vi "Serial Read.vi"(9 "Timeout (ms)":i32, 10 "Number of Bytes to Read":u32, 11 "IO Cluster In":T1={"Error"={"status"=FALSE, "code"=0, "source"=""}, "Encoder Calibration Values"=[22, 216], "Update Calibration"=FALSE, "JPEG Resolutions"=3, "Raw Resolutions"=1, "Image Mode"=enum."RAW Gray Scale", "FPGA Ref"=refnum} {"JPEG Resolutions" items=["160x128"=3, "320x240"=5, "640x480"=7]; "Raw Resolutions" items=["80x60"=1, "160x120"=3, "128x128"=9, "128x96"=11]}) -> (1 "Data Valid":bool, 2 "Data":u8[](array[numeric]), 3 "IO Cluster Out":T1={"Error"={"status"=FALSE, "code"=0, "source"=""}, "Encoder Calibration Values"=[22, 216], "Update Calibration"=FALSE, "JPEG Resolutions"=3, "Raw Resolutions"=1, "Image Mode"=enum."RAW Gray Scale", "FPGA Ref"=refnum} {"JPEG Resolutions" items=["160x128"=3, "320x240"=5, "640x480"=7]; "Raw Resolutions" items=["80x60"=1, "160x120"=3, "128x128"=9, "128x96"=11]}, 4 "Framing Error":bool, 6 "Bytes in Buffer":u32)   [LabVIEW 2019]
uses:
  QNET MS IO Cluster.ctl
  <vilib>/Utility/error.llb/Error Cluster From Error Code.vi
  <vilib>/rvi/errors/niLvFpgaAdjustHostInterfaceError.vi
  <vilib>/rvi/interface/nirviMethod/nirviMethod.xnode
  <vilib>/rvi/interface/nirviReadWriteControl/nirviReadWriteControl.xnode
  <vilib>/FPGAPlugInAG/Dynamic/niLvFpga_ReadFifo_Dynamic.vi
  <vilib>/rvi/errors/niLvFpgaMergeErrorWithErrorCode.vi
  NiFpgaLv.dll
  <vilib>/rvi/interface/Simulation/niFpgaSimulationCallBeginRW.vi
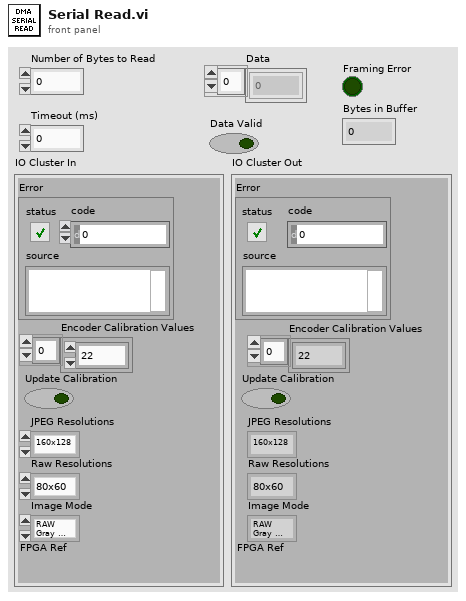
[diagram p1: front panel]
types:
  T1 = typedef "QNET MS IO Cluster.ctl" = cluster{"Error":errorcluster, "Encoder Calibration Values":i32[], "Update Calibration":bool, "JPEG Resolutions":u16, "Raw Resolutions":u16, "Image Mode":enum16{"RAW RGB", "RAW Gray Scale", "JPEG"}, "FPGA Ref":refnum<k20>}
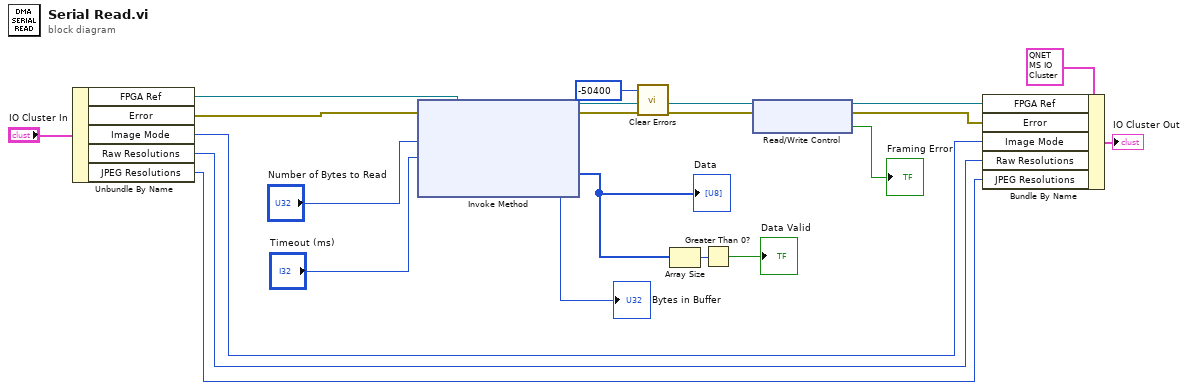
[diagram p0: block diagram]
diagram:
  n1 = Unbundle By Name("IO Cluster In") -> ("FPGA Ref"=w13:refnum<k20>, "Error"=w12:errorcluster, "Image Mode"=w9:enum16{"RAW RGB", "RAW Gray Scale", "JPEG"}, "Raw Resolutions"=w8:u16, "JPEG Resolutions"=w7:u16)
  n2 = xnode "Invoke Method"("FPGA VI引用输入"=w13, "错误输入"=w12, "Number of Elements"="Number of Bytes to Read", "Timeout (ms)"="Timeout (ms)") -> ("FPGA VI引用输出"=w18:refnum<k20>, "错误输出"=w6:errorcluster, "Data"=w21:u8[], "Elements Remaining"=→"Bytes in Buffer":u32)
  "Data" <- w21
  n3 = call <vilib>:"Clear Errors.vi"("error in (no error)"=w6, "specific error code to clear (0: all)"=-50400 ("code")) -> ("error out"=w5:errorcluster)  [unwired: 4 in, 1 out]
  n4 = Array Size(array=w21) -> (size(s)=w19:i32)
  n5 = Greater Than 0?(x=w19) -> (x > 0?=→"Data Valid":bool)
  n6 = xnode "Read/Write Control"("FPGA VI引用输入"=w18, "错误输入"=w5) -> ("FPGA VI引用输出"=w11:refnum<k20>, "错误输出"=w10:errorcluster, "Framing Error"=→"Framing Error":bool)
  n7 = Bundle By Name(cluster=T1 {"Error"={"status"=FALSE, "code"=0, "source"=""}, "Encoder Calibration Values"=[22, 216], "Update Calibration"=FALSE, "JPEG Resolutions"=3, "Raw Resolutions"=1, "Image Mode"=enum."RAW Gray Scale", "FPGA Ref"=refnum} ("IO Cluster In"), "FPGA Ref"=w11, "Error"=w10, "Image Mode"=w9, "Raw Resolutions"=w8, "JPEG Resolutions"=w7) -> (→"IO Cluster Out":T1)
